vi "CH2_Tx.vi"() -> ()   [LabVIEW 2018]
uses:
  Stream/Stream.lvclass
  RxTx/RxTx.lvclass
panel:
  in  "RxTx.lvclass":refnum<class "RxTx.lvclass">
  in  "Stream.lvclass":refnum<class "Stream.lvclass">
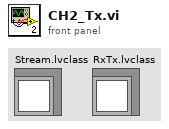
[diagram p1: front panel]
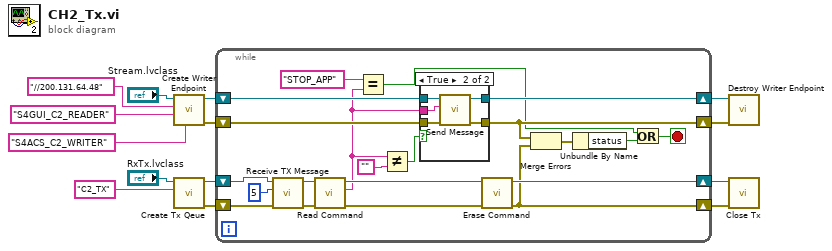
[diagram p0: block diagram]
diagram:
  n1 = call "Create Writer Endpoint.vi"("writer name"="S4ACS_C2_WRITER" ("reader name"), "reader name"="S4GUI_C2_READER", "IP"="//200.131.64.48" ("Reader Name"), "Stream in"="Stream.lvclass") -> ("error out"=w5:errorcluster, "Stream out"=w7:refnum<class "Stream.lvclass">)  [unwired: 6 in]
  n2 = call "Create Tx Qeue.vi"("Writer Name"="C2_TX" ("Reader Name"), "RxTx in"="RxTx.lvclass") -> ("error out"=w12:errorcluster, "RxTx out"=w13:refnum<class "RxTx.lvclass">)  [unwired: 8 in]
  n3 = while {
    shift-right: [w26] -> w1
    shift-left: w5 -> [w28]
    shift-right: [w27] -> w14
    shift-left: w7 -> [w29]
    shift-right: [w20] -> w8
    shift-left: w12 -> [w30]
    shift-right: [w22] -> w9
    shift-left: w13 -> [w31]
    stop <- w19 stop-if-true
    n4 = call "Receive TX Message.vi"("error in (no error)"=w30, "timeout in ms"=5, "RxTx in"=w31) -> ("error out"=w34:errorcluster, "RxTx out"=w33:refnum<class "RxTx.lvclass">)  [unwired: 7 in]
    n5 = call "Read Command.vi"("error in (no error)"=w34, "RxTx in"=w33) -> ("error out"=w21:errorcluster, "Message"=w15:string, "RxTx out"=w23:refnum<class "RxTx.lvclass">)  [unwired: 7 in]
    n6 = Equal?(x="STOP_APP" ("Reader Name"), y=w15) -> (x = y?=w17:bool)
    n7 = Not Equal?(x=w15, y="") -> (x != y?=w25:bool)
    n8 = case shown="True" w25 {
      tunnel: w29 -> [w37 w42]
      tunnel: w28 -> [w36 w41]
      tunnel: [w37 w40] -> w27
      tunnel: w15 -> [_ w39]
      tunnel: [w36 w38] -> w26
      frame False {
      }
      frame True {
        n9 = call "Send Message.vi"("error in (no error)"=w41, "Message"=w39, "Stream in"=w42) -> ("error out"=w38:errorcluster, "Stream out"=w40:refnum<class "Stream.lvclass">)  [unwired: 7 in]
      }
    }
    n10 = call "Erase Command.vi"("error in (no error)"=w21, "RxTx in"=w23) -> ("error out"=w20:errorcluster, "RxTx out"=w22:refnum<class "RxTx.lvclass">)  [unwired: 8 in]
    n11 = Merge Errors(w26, w20) -> (w35:errorcluster)
    n12 = Unbundle By Name(w35) -> ("status"=w18:bool)
    n13 = Or(x=w17, y=w18) -> (x .or. y?=w19:bool)
  }
  n14 = call "Destroy Writer Endpoint.vi"("error in (no error)"=w1, "Stream in"=w14) -> ()  [unwired: 8 in, 2 out]
  n15 = call "Close Tx.vi"("error in (no error)"=w8, "RxTx in"=w9) -> ()  [unwired: 8 in, 2 out]
